vi "interleave array around index.vi"(1 "index":i32, 2 "Array in":cluster{"x":i16, "y":i16}[](array[cluster])) -> (0 "Array out":cluster{"x":i16, "y":i16}[](array[cluster]))   [LabVIEW 2009]
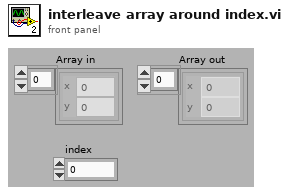
[diagram p1: front panel]
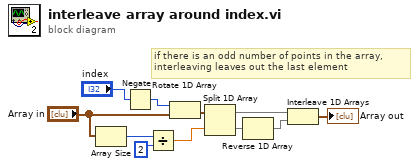
[diagram p0: block diagram]
diagram:
  # "if there is an odd number of points in the array, interleaving leaves out the last element"
  n1 = Array Size(array="Array in") -> (size(s)=w8:i32)
  n2 = Negate(x="index") -> (-x=w1:i32)
  n3 = Divide(x=w8, y=2) -> (x/y=w10:dbl)
  n4 = Rotate 1D Array(1:"Array in", 2:w1) -> (0:w9:cluster{"x":i16, "y":i16}[])
  n5 = Split 1D Array(array=w9, index=w10) -> (first subarray=w4:cluster{"x":i16, "y":i16}[], second subarray=w5:cluster{"x":i16, "y":i16}[])
  n6 = Reverse 1D Array(array=w5) -> (reversed array=w3:cluster{"x":i16, "y":i16}[])
  n7 = Interleave 1D Arrays(w4, w3) -> (→"Array out":cluster{"x":i16, "y":i16}[])
